vi "Read Thermistor T.vi"(8 "error in (no error)":errorcluster, 11 "cCRDS Data in":refnum<class "cCRDS Data.lvclass">=refnum) -> (0 "error out":errorcluster, 2 "Thermistor T":sgl[](array[numeric]), 3 "cCRDS Data out":refnum<class "cCRDS Data.lvclass">)   [LabVIEW 2015, in "cCRDS Data.lvclass"]
uses:
  cCRDS Data.lvclass
  cCRDS Data.lvclass/cCRDS Data.ctl
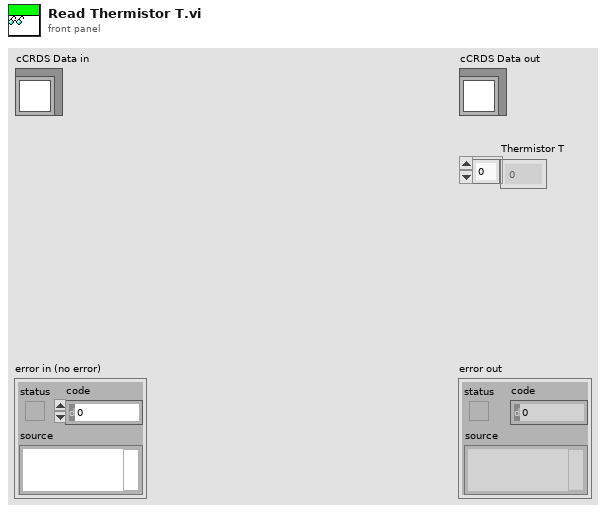
[diagram p1: front panel]
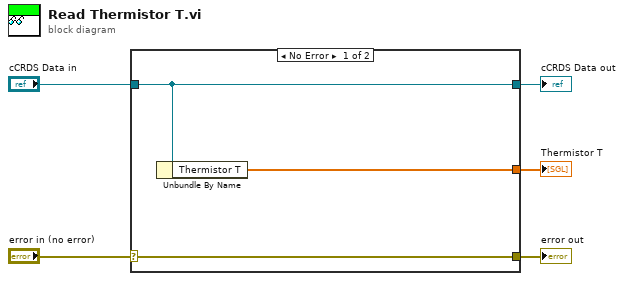
[diagram p0: block diagram]
diagram:
  n1 = case shown="No Error" "error in (no error)" {
    selector: "error in (no error)" -> [w8 w9]
    tunnel: [w8 w9] -> w4
    tunnel: [w7 w10] -> w2
    tunnel: "cCRDS Data in" -> [w7 w10]
    tunnel: [w6 _] -> w1
    frame No Error {
      n2 = Unbundle By Name(w7) -> ("Thermistor T"=w6:sgl[])
    }
    frame Error {
    }
  }
  "error out" <- w4
  "cCRDS Data out" <- w2
  "Thermistor T" <- w1
